vi "Save VI with XML Heaps.vi"(8 "error in (no error)":errorcluster, 9 "Heap Save Format (1=XML)":T1=1 items=["Off", "XML", "Binary", "Verbose Tagged Text", "Binary2"], 10 "VI Path (temporary file)":path=path "", 11 "VI Refnum In":refnum<vi>) -> (0 "error out":errorcluster, 2 "VI Path out":path, 3 "VI Refnum Out":refnum<vi>)   [LabVIEW 2023]
uses:
  CTLs/Heap Save Format.ctl
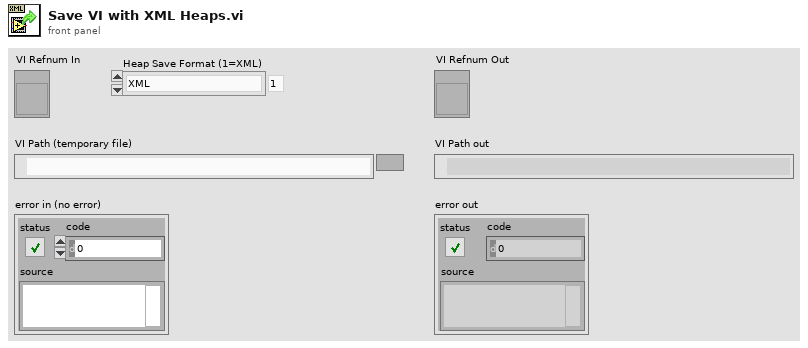
[diagram p1: front panel]
types:
  T1 = typedef "Heap Save Format.ctl" = u16
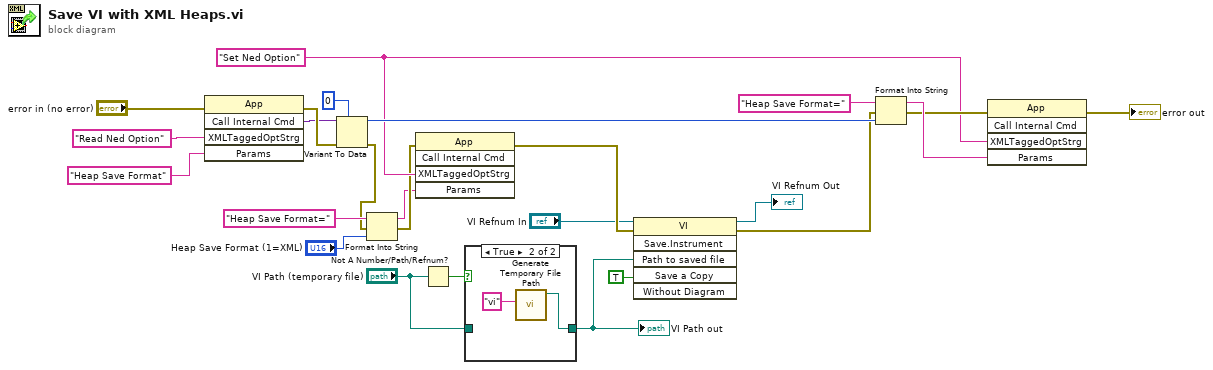
[diagram p0: block diagram]
diagram:
  w16 = "Set Ned Option" ("Command Name")
  n1 = invoke class="App" method="Call Internal Cmd"(error in="error in (no error)", "XMLTaggedOptStrg"="Read Ned Option" ("Command Name"), "Params"="Heap Save Format") -> (error out=w25:errorcluster, "CallInternalCmd"=w22:variant)  [unwired: 2 in, 3 out]
  n2 = Variant To Data(error in=w25, type=0, Variant=w22) -> (data=w19:i32, error out=w3:errorcluster)
  n3 = Format Into String(initial string="Heap Save Format=", error in=w3, "Heap Save Format (1=XML)") -> (resulting string=w1:string, error out=w2:errorcluster)  [unwired: 1 in]
  n4 = invoke class="App" method="Call Internal Cmd"(error in=w2, "XMLTaggedOptStrg"=w16, "Params"=w1) -> (error out=w15:errorcluster)  [unwired: 2 in, 4 out]
  n5 = Not A Number/Path/Refnum?(number/path/refnum="VI Path (temporary file)") -> (NaN/Path/Refnum?=w9:bool)
  n6 = case shown="True" w9 {
    tunnel: [w26 w28] -> w7
    tunnel: "VI Path (temporary file)" -> [w26 _]
    frame False {
    }
    frame True {
      n7 = call <vilib>:"Generate Temporary File Path.vi"("Temporary File Extension (tmp)"="vi") -> ("Unique Temporary File Path"=w28:path)  [unwired: 9 in, 1 out]
    }
  }
  "VI Path out" <- w7
  n8 = invoke class="VI" method="Save.Instrument"(reference="VI Refnum In", error in=w15, "Path to saved file"=w7, "Save a Copy"=TRUE) -> (reference out=→"VI Refnum Out":refnum<vi>, error out=w14:errorcluster)  [unwired: 2 in, 4 out]
  n9 = Format Into String(initial string="Heap Save Format=", error in=w14, w19) -> (resulting string=w18:string, error out=w17:errorcluster)  [unwired: 1 in]
  n10 = invoke class="App" method="Call Internal Cmd"(error in=w17, "XMLTaggedOptStrg"=w16, "Params"=w18) -> (error out=→"error out":errorcluster)  [unwired: 2 in, 4 out]
